vi "oa_Get Reference Data in Resampled Waveform.vi"(5 "reset? (True)":bool=TRUE, 6 "select reference data":T1(ring), 7 "# of revs in reference data":i32=1, 8 "error in (no error)":errorcluster, 9 "last index":i32=1, 10 "pulse per rev":dbl=1.0 format="%.2p", 11 "Y":dbl[](array[numeric]) format="%.2f") -> (0 "error out":errorcluster, 1 "last index out":i32=1, 3 "reference data":dbl[](array[numeric]) format="%.2f")   [LabVIEW 2017, in "SoundVib_RefDataProcess.lvlib"]
uses:
  <vilib>/addons/Sound and Vibration/Order Analysis/Referece Data Processing/SoundVib_RefDataProcess.lvlib
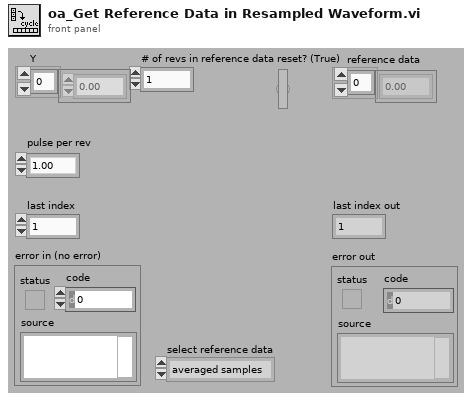
[diagram p1: front panel]
types:
  T1 = enum16{"averaged samples", "initial samples", "final samples"}
  T2 = cluster{"is warning? (False)":bool, "error code (0)":i32, "error message (\"\")":string}
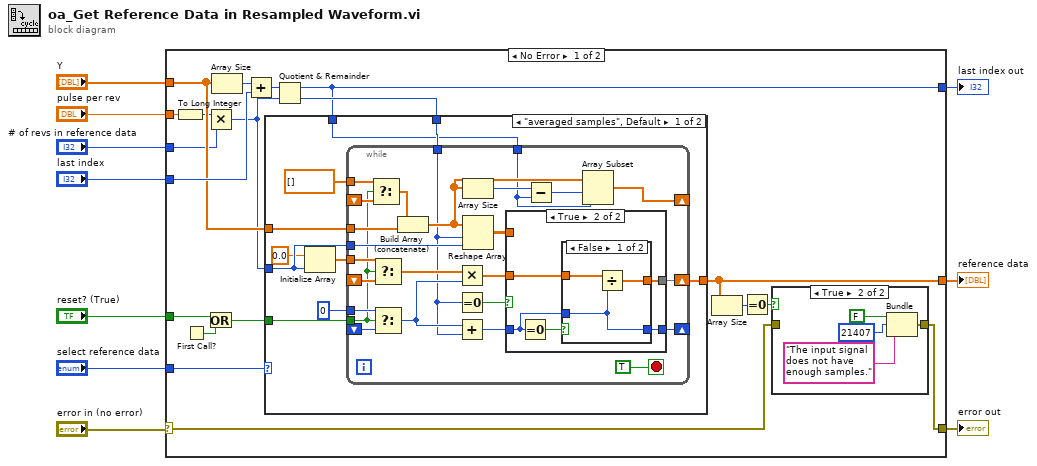
[diagram p0: block diagram]
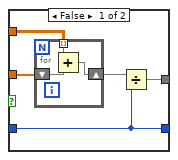
[diagram p3: hidden frame]
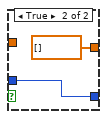
[diagram p4: hidden frame]
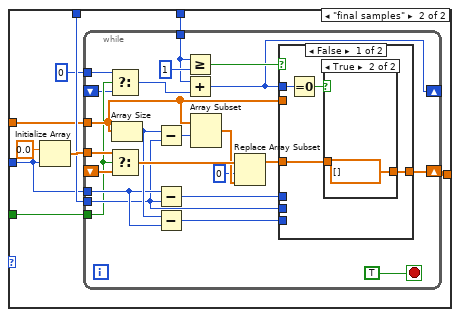
[diagram p5: hidden frame]
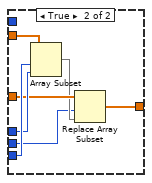
[diagram p7: hidden frame]
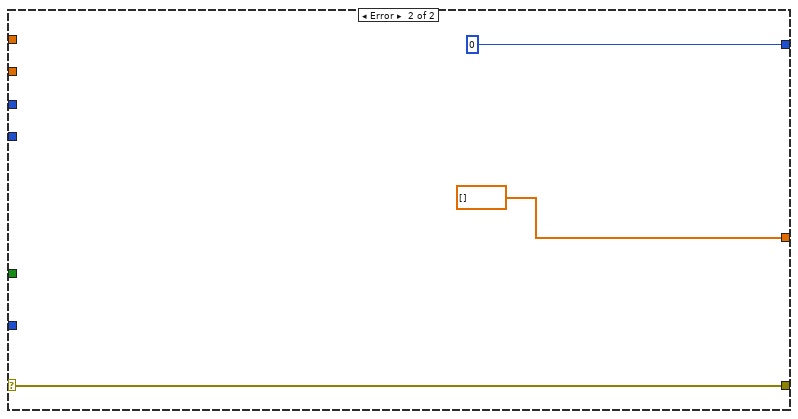
[diagram p8: hidden frame]
diagram:
  n1 = case shown="No Error" "error in (no error)" {
    selector: "error in (no error)" -> [w12 w135]
    tunnel: [w11 w135] -> w9
    tunnel: "select reference data" -> [w29 _]
    tunnel: "Y" -> [w25 _]
    tunnel: "last index" -> [w26 _]
    tunnel: [w23 0] -> w5
    tunnel: "reset? (True)" -> [w22 _]
    tunnel: [w15 dbl[] []] -> w3
    tunnel: "# of revs in reference data" -> [w18 _]
    tunnel: "pulse per rev" -> [w17 _]
    frame No Error {
      n2 = To Long Integer(number=w17) -> (32bit integer=w19:i32)
      n3 = First Call?() -> (First Call?: T/F=w21:bool)
      n4 = Multiply(x=w19, y=w18) -> (x*y=w16:i32)
      n5 = Or(x=w22, y=w21) -> (x .or. y?=w20:bool)
      n6 = Array Size(array=w25) -> (size(s)=w27:i32)
      n7 = Add(x=w27, y=w26) -> (x+y=w28:i32)
      n8 = Quotient & Remainder(x=w28, y=w16) -> (x-y*floor(x/y)=w23:i32, floor(x/y)=w24:i32)
      n9 = case shown="\"averaged samples\", Default" w29 {
        tunnel: w20 -> [w44 w95]
        tunnel: w25 -> [w37 w90]
        tunnel: w24 -> [w43 w92]
        tunnel: [w41 w93] -> w15
        tunnel: w16 -> [w39 w89]
        tunnel: w23 -> [w35 w91]
        frame "averaged samples", Default {
          n10 = Initialize Array(0.0 ("element"), w39) -> (w40:dbl[])
          n11 = while {
            tunnel: w44 -> [w56]
            shift-right: [w47] -> w41
            shift-left: _ -> [w68]
            tunnel: w40 -> [w67]
            tunnel: w43 -> [w49]
            shift-right: [w45] -> _
            shift-left: _ -> [w65]
            tunnel: 0 -> [w64]
            tunnel: w39 -> [w61]
            shift-right: [w50] -> _
            shift-left: _ -> [w58]
            tunnel: w37 -> [w59]
            tunnel: dbl[] [] ("initialized array") -> [w55]
            tunnel: w35 -> [w51]
            stop <- TRUE stop-if-true
            n12 = Select(t=w55, s=w56, f=w58) -> (s? t:f=w57:dbl[])
            n13 = Select(t=w67, s=w56, f=w68) -> (s? t:f=w63:dbl[])
            n14 = Select(t=w64, s=w56, f=w65) -> (s? t:f=w60:i32)
            n15 = Build Array (concatenate)(w57, w59) -> (w54:dbl[])
            n16 = Multiply(x=w63, y=w60) -> (x*y=w62:dbl[])
            n17 = Equal To 0?(x=w49) -> (x = 0?=w48:bool)
            n18 = Add(x=w60, y=w49) -> (x+y=w46:i32)
            n19 = Array Size(array=w54) -> (size(s)=w53:i32)
            n20 = Reshape Array(w54, w49, w61) -> (w66:dbl[][])
            n21 = case shown="True" w48 {
              tunnel: w66 -> [w74 _]
              tunnel: w62 -> [w73 w80]
              tunnel: [w71 w81] -> w47
              tunnel: w46 -> [w70 w79]
              tunnel: [w70 w78] -> w45
              frame False {
                n22 = for {
                  tunnel: w74 -> [w77] mode=indexing
                  shift-right: [w75] -> w72
                  shift-left: w73 -> [w76]
                  n23 = Add(x=w77, y=w76) -> (x+y=w75:dbl[])
                }
                n24 = Divide(x=w72, y=w70) -> (x/y=w71:dbl[])
              }
              frame True {
                n25 = Equal To 0?(x=w79) -> (x = 0?=w82:bool)
                n26 = case shown="False" w82 {
                  tunnel: [w84 dbl[] []] -> w81
                  tunnel: w80 -> [w85 _]
                  tunnel: w79 -> [w83 w87]
                  tunnel: [w83 w87] -> w78
                  frame False {
                    n27 = Divide(x=w85, y=w83) -> (x/y=w84:dbl[])
                  }
                  frame True {
                  }
                }
              }
            }
            n28 = Subtract(x=w53, y=w51) -> (x-y=w52:i32)
            n29 = Array Subset(array=w54, index=w52, length=w51) -> (w50:dbl[])
          }
        }
        frame "final samples" {
          n30 = Initialize Array(0.0 ("element"), w89) -> (w94:dbl[])
          n31 = while {
            tunnel: w95 -> [w102]
            tunnel: w94 -> [w119]
            shift-right: [w111] -> w93
            shift-left: _ -> [w118]
            tunnel: w92 -> [w99]
            tunnel: w91 -> [w103]
            tunnel: w90 -> [w110]
            tunnel: w89 -> [w108]
            shift-right: [w97] -> _
            shift-left: _ -> [w98]
            tunnel: 0 ("y") -> [w101]
            stop <- TRUE stop-if-true
            n32 = Select(t=w101, s=w102, f=w98) -> (s? t:f=w100:i32)
            n33 = Select(t=w119, s=w102, f=w118) -> (s? t:f=w115:dbl[])
            n34 = Array Size(array=w110) -> (size(s)=w109:i32)
            n35 = Subtract(x=w109, y=w103) -> (x-y=w106:i32)
            n36 = Subtract(x=w108, y=w103) -> (x-y=w105:i32)
            n37 = Subtract(x=w109, y=w108) -> (x-y=w107:i32)
            n38 = Greater Or Equal?(x=w99, y=1) -> (x >= y?=w113:bool)
            n39 = Add(x=w99, y=w100) -> (x+y=w97:i32)
            n40 = Array Subset(array=w110, index=w106) -> (w114:dbl[])  [unwired: 1 in]
            n41 = Replace Array Subset(array=w115, new element=w114, index=0) -> (w112:dbl[])
            n42 = case shown="False" w113 {
              tunnel: w112 -> [w121 w128]
              tunnel: [w120 w129] -> w111
              tunnel: w110 -> [_ w132]
              tunnel: w107 -> [_ w131]
              tunnel: w105 -> [_ w130]
              tunnel: w103 -> [_ w126]
              tunnel: w97 -> [w123 _]
              frame False {
                n43 = Equal To 0?(x=w123) -> (x = 0?=w122:bool)
                n44 = case shown="True" w122 {
                  tunnel: w121 -> [w124 _]
                  tunnel: [w124 dbl[] []] -> w120
                  frame False {
                  }
                  frame True {
                  }
                }
              }
              frame True {
                n45 = Array Subset(array=w132, index=w131, length=w130) -> (w127:dbl[])
                n46 = Replace Array Subset(array=w128, new element=w127, index=w126) -> (w129:dbl[])
              }
            }
          }
        }
      }
      n47 = Array Size(array=w15) -> (size(s)=w14:i32)
      n48 = Equal To 0?(x=w14) -> (x = 0?=w13:bool)
      n49 = case shown="True" w13 {
        tunnel: w12 -> [w30 _]
        tunnel: [w30 w31] -> w11
        frame False {
        }
        frame True {
          n50 = Bundle("is warning? (False)"=FALSE, "error code (0)"=21407, "error message (\"\")"="The input signal does not have enough samples." ("error message (\"\")")) -> (w31:T2)  [unwired: 1 in]
        }
      }
    }
    frame Error {
    }
  }
  "error out" <- w9
  "last index out" <- w5
  "reference data" <- w3
